vi "Cypher XY LVDT Parameters_MFP3D_Lucy.vi"() -> ()   [LabVIEW 2013]
panel:
  in  "Cypher YLVDT Offset":dbl=0.07
  in  "Cypher XLVDT Offset":dbl=-0.63
  in  "Cypher YLVDT Sens":dbl=7.0428e-06
  in  "Cypher XLVDT Sens":dbl=7.4643e-06
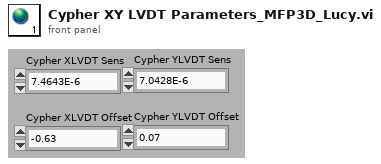
[diagram p1: front panel]
diagram:
